vi "Quaternion to Rotation Matrix.vi"(1 "quaternion":T2) -> (0 "rotation matrix":T1)   [LabVIEW 2017, in "NI_Kinematics.lvlib"]
doc: "Converts a unit quaternion to the corresponding <B>rotation matrix</B>."
uses:
  <vilib>/robotics/Kinematics/NI_Kinematics.lvlib
  <vilib>/robotics/Kinematics/Quaternion.ctl
  <vilib>/Analysis/Matrix/Datatypes/RealMatrix.ctl
  <vilib>/Analysis/baseanly.llb/Real Outer Product.vi
  <vilib>/Analysis/Matrix/Numeric/Add/Add - RM,RM.vi
  <vilib>/Analysis/Matrix/Numeric/Multiply/Multiply - RM,R.vi
  <vilib>/Analysis/Matrix/Numeric/Multiply/Multiply - R,RM.vi
  <vilib>/Analysis/NI_AALBase.lvlib
  <vilib>/Analysis/Matrix/NI_Matrix.lvlib
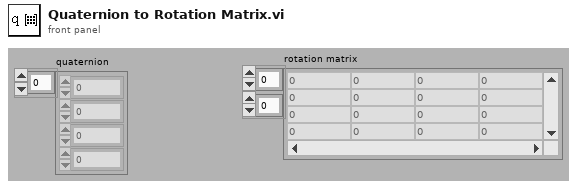
[diagram p1: front panel]
types:
  T1 = typedef "NI_Matrix.lvlib/RealMatrix.ctl" = dbl[][]
  T2 = typedef "NI_Kinematics.lvlib/Quaternion.ctl" = dbl[]
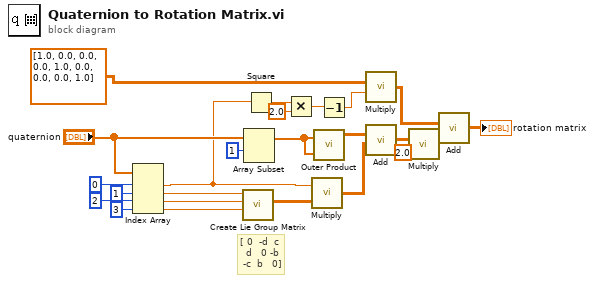
[diagram p0: block diagram]
diagram:
  # "[ 0  -d  c\n  d   0 -b\n -c  b   0]"
  n1 = Index Array(array="quaternion", index #1=0 ("index"), index #2=1 ("index"), index #3=2 ("index"), index #4=3 ("index")) -> (element #1=w3:dbl, element #2=w13:dbl, element #3=w12:dbl, element #4=w11:dbl)
  n2 = call <vilib>:"Create Lie Group Matrix.vi"("z"=w11, "y"=w12, "x"=w13) -> ("real matrix"=w10:T1)  [unwired: 8 in]
  n3 = Array Subset(array="quaternion", index=1) -> (w8:T2)  [unwired: 1 in]
  n4 = Square(x=w3) -> (x^2=w4:dbl)
  n5 = Multiply(x=w4, y=2.0) -> (x*y=w6:dbl)
  n6 = call-poly <vilib>:"Multiply.vi"("Real Matrix A"=w10, "Real Scalar c"=w3) -> ("c * A"=w22:T1)
  n7 = call-poly <vilib>:"Outer Product.vi"("Y Vector"=w8, "X Vector"=w8) -> ("Outer Product"=w21:T1)  [unwired: 1 out]
  n8 = Decrement(x=w6) -> (x-1=w2:dbl)
  n9 = call-poly <vilib>:"Multiply.vi"("Real Scalar c"=w2, "Real Matrix A"=T1 [[1.0, 0.0, 0.0], [0.0, 1.0, 0.0], [0.0, 0.0, 1.0]] ("Special Matrix")) -> ("A * c"=w19:T1)
  n10 = call-poly <vilib>:"Add.vi"("Real Matrix B"=w22, "Real Matrix A"=w21) -> ("A + B"=w20:T1)
  n11 = call-poly <vilib>:"Multiply.vi"("Real Scalar c"=2.0 ("dimension size"), "Real Matrix A"=w20) -> ("A * c"=w18:T1)
  n12 = call-poly <vilib>:"Add.vi"("Real Matrix B"=w18, "Real Matrix A"=w19) -> ("A + B"=→"rotation matrix":T1)
